vi "Accumulator.vi"(9 "Reset Accumulator":bool, 10 "Delta Angle":dbl format="%#_13g") -> (2 "Combined Angle":dbl)   [LabVIEW 2019]
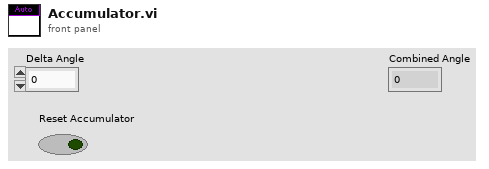
[diagram p1: front panel]
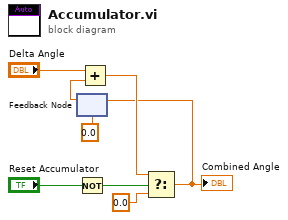
[diagram p0: block diagram]
diagram:
  n1 = feedback #1(0.0) -> (w8:dbl)
  n2 = Not(x="Reset Accumulator") -> (.not. x?=w1:bool)
  n3 = Add(x="Delta Angle", y=w8) -> (x+y=w4:dbl)
  n4 = Select(t=w4, s=w1, f=0.0 ("t")) -> (s? t:f=w3:dbl)
  "Combined Angle" <- w3
  n5 = feedback-in #1(w3) -> ()
